vi "Configure DAQmx Task.vi"(8 "error in (no error)":errorcluster, 9 "DAQmx Timing Settings In":T2, 10 "Trigger Settings In":T1={"Trigger Type"=enum."No Trigger", "Digital Start"={"Source"="", "Digital Start Trigger Edge"=0}, "Digital Pause"={"Source"="", "Digital Pause Trigger Pause When"=0}, "Digital Reference"={"Source"="", "Digital Start Trigger Edge"=0, "Digital Reference Pretrigger Samples"=0}, "Analog Start"={"Source"="", "Analog Slope"=0, "Analog Start Trigger Hysteresis"=0.0, "Analog Start Trigger Level"=0.0}, "Analog Pause"={"Source"="", "Analog Start Trigger Level"=0.0, "Analog Pause Trigger Pause When"=10093}, "Analog Reference"={"Source"="", "Slope"=10280, "Pretrigger Samples"=0, "Level"=0.0}, "Time Start"={"Select Time\nManually"=FALSE, "When"=timestamp(0 s since 1904-01-01)}} caption="Some parts are hidden" {"Time Start"."When" format="%<%x %.3X>T"; "Analog Reference"."Level" format="%0.2f"; "Analog Reference"."Slope" items=["Rising"=10280, "Falling"=10171]; "Analog Pause"."Analog Pause Trigger Pause When" items=["Above Level"=10093, "Below Level"=10107]; "Analog Pause"."Analog Start Trigger Level" format="%0.2f"; "Analog Start"."Analog Start Trigger Level" format="%0.2f"; "Analog Start"."Analog Start Trigger Hysteresis" format="%.2f"; "Analog Start"."Analog Slope" items=["Rising"=10280, "Falling"=10171]; "Digital Reference"."Digital Start Trigger Edge" items=["Rising"=10280, "Falling"=10171]; "Digital Pause"."Digital Pause Trigger Pause When" items=["High"=10192, "Low"=10214]; "Digital Start"."Digital Start Trigger Edge" items=["Rising"=10280, "Falling"=10171]}, 11 "HW Refnum In":string) -> (0 "error out":errorcluster, 1 "Trigger Settings Out":T1={"Trigger Type"=enum."No Trigger", "Digital Start"={"Source"="", "Digital Start Trigger Edge"=0}, "Digital Pause"={"Source"="", "Digital Pause Trigger Pause When"=0}, "Digital Reference"={"Source"="", "Digital Start Trigger Edge"=0, "Digital Reference Pretrigger Samples"=0}, "Analog Start"={"Source"="", "Analog Slope"=0, "Analog Start Trigger Hysteresis"=0.0, "Analog Start Trigger Level"=0.0}, "Analog Pause"={"Source"="", "Analog Start Trigger Level"=0.0, "Analog Pause Trigger Pause When"=10093}, "Analog Reference"={"Source"="", "Slope"=10280, "Pretrigger Samples"=0, "Level"=0.0}, "Time Start"={"Select Time\nManually"=FALSE, "When"=timestamp(0 s since 1904-01-01)}} caption="Some parts are hidden" {"Time Start"."When" format="%<%x %.3X>T"; "Analog Reference"."Level" format="%0.2f"; "Analog Reference"."Slope" items=["Rising"=10280, "Falling"=10171]; "Analog Pause"."Analog Pause Trigger Pause When" items=["Above Level"=10093, "Below Level"=10107]; "Analog Pause"."Analog Start Trigger Level" format="%0.2f"; "Analog Start"."Analog Start Trigger Level" format="%0.2f"; "Analog Start"."Analog Start Trigger Hysteresis" format="%.2f"; "Analog Start"."Analog Slope" items=["Rising"=10280, "Falling"=10171]; "Digital Reference"."Digital Start Trigger Edge" items=["Rising"=10280, "Falling"=10171]; "Digital Pause"."Digital Pause Trigger Pause When" items=["High"=10192, "Low"=10214]; "Digital Start"."Digital Start Trigger Edge" items=["Rising"=10280, "Falling"=10171]}, 2 "DAQmx Timing Settings Out":T2, 3 "HW Refnum Out":string)   [LabVIEW 2020, in "Acquisition.lvlib"]
uses:
  Acquisition.lvlib
  Settings Editor/DAQmx Trigger Settings--cluster.ctl
  <vilib>/DAQmx/configure/timing.llb/DAQmx Timing (Sample Clock).vi
  <vilib>/DAQmx/configure/trigger.llb/DAQmx Start Trigger (Digital Edge).vi
  <vilib>/DAQmx/configure/trigger.llb/DAQmx Start Trigger (Time).vi
  <vilib>/DAQmx/configure/trigger.llb/DAQmx Start Trigger (Analog Edge).vi
  <vilib>/DAQmx/configure/trigger.llb/DAQmx Reference Trigger (Digital Edge).vi
  <vilib>/DAQmx/configure/trigger.llb/DAQmx Reference Trigger (Analog Edge).vi
  <resource>/objmgr/daqmx.rc
  Settings Editor/Settings Editor.lvlib
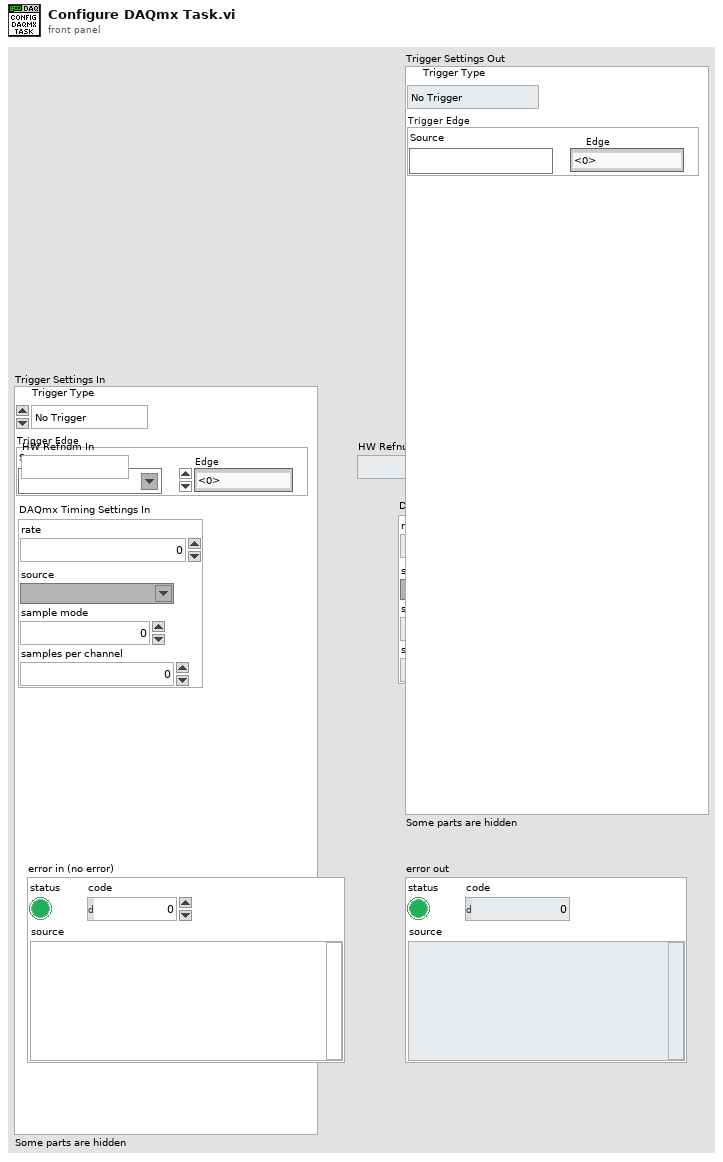
[diagram p1: front panel]
types:
  T1 = typedef "Settings Editor.lvlib/DAQmx Trigger Settings--cluster.ctl" = cluster{"Trigger Type":enum32{"No Trigger", "Digital Start", "Digital Pause", "Digital Reference", "Analog Start", "Analog Pause", "Analog Reference", "Time Start"}, "Digital Start":cluster{"Source":tag, "Digital Start Trigger Edge":i32}, "Digital Pause":cluster{"Source":tag, "Digital Pause Trigger Pause When":i32}, "Digital Reference":cluster{"Source":tag, "Digital Start Trigger Edge":i32, "Digital Reference Pretrigger Samples":u32}, "Analog Start":cluster{"Source":string, "Analog Slope":i32, "Analog Start Trigger Hysteresis":dbl, "Analog Start Trigger Level":dbl}, "Analog Pause":cluster{"Source":string, "Analog Start Trigger Level":dbl, "Analog Pause Trigger Pause When":i32}, "Analog Reference":cluster{"Source":string, "Slope":i32, "Pretrigger Samples":u32, "Level":dbl}, "Time Start":cluster{"Select Time\nManually":bool, "When":timestamp}}
  T2 = cluster{"rate":dbl, "source":tag, "sample mode":i32, "samples per channel":i32}
  T3 = enum32{"No Trigger", "Digital Start", "Digital Pause", "Digital Reference", "Analog Start", "Analog Pause", "Analog Reference", "Time Start"}
  T4 = cluster{"Source":tag, "Digital Start Trigger Edge":i32}
  T5 = cluster{"Select Time\nManually":bool, "When":timestamp}
  T6 = cluster{"Source":string, "Analog Slope":i32, "Analog Start Trigger Hysteresis":dbl, "Analog Start Trigger Level":dbl}
  T7 = cluster{"Source":tag, "Digital Start Trigger Edge":i32, "Digital Reference Pretrigger Samples":u32}
  T8 = cluster{"Source":string, "Slope":i32, "Pretrigger Samples":u32, "Level":dbl}
  T9 = cluster{"Source":tag, "Digital Pause Trigger Pause When":i32}
  T10 = cluster{"Source":string, "Analog Start Trigger Level":dbl, "Analog Pause Trigger Pause When":i32}
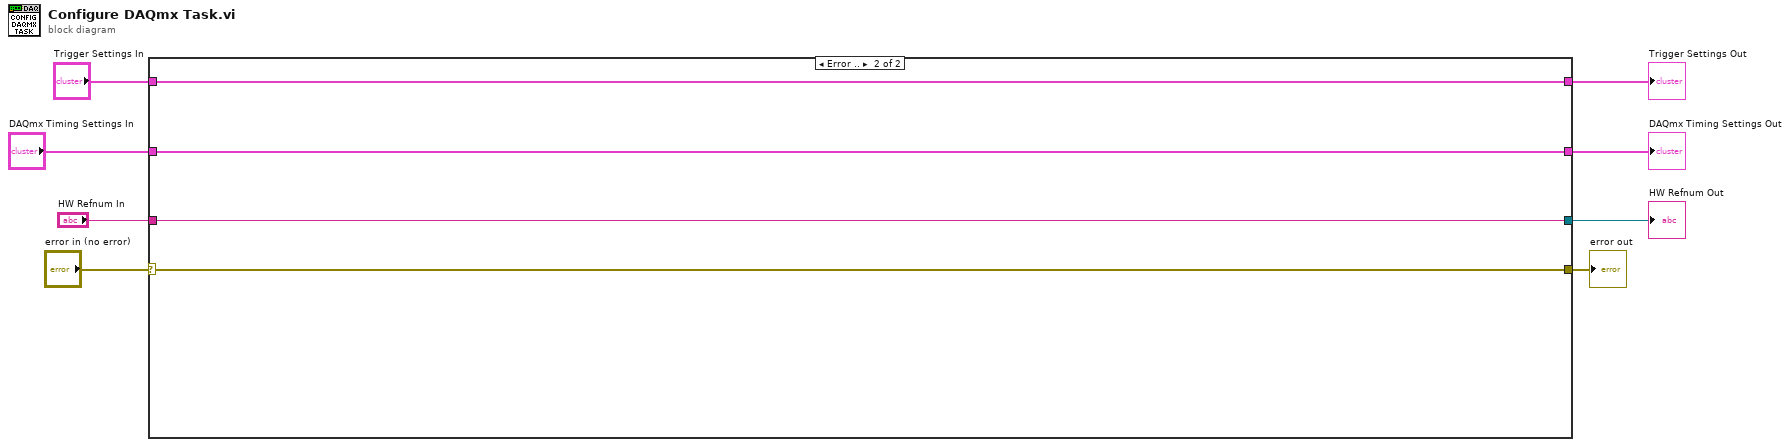
[diagram p0: block diagram]
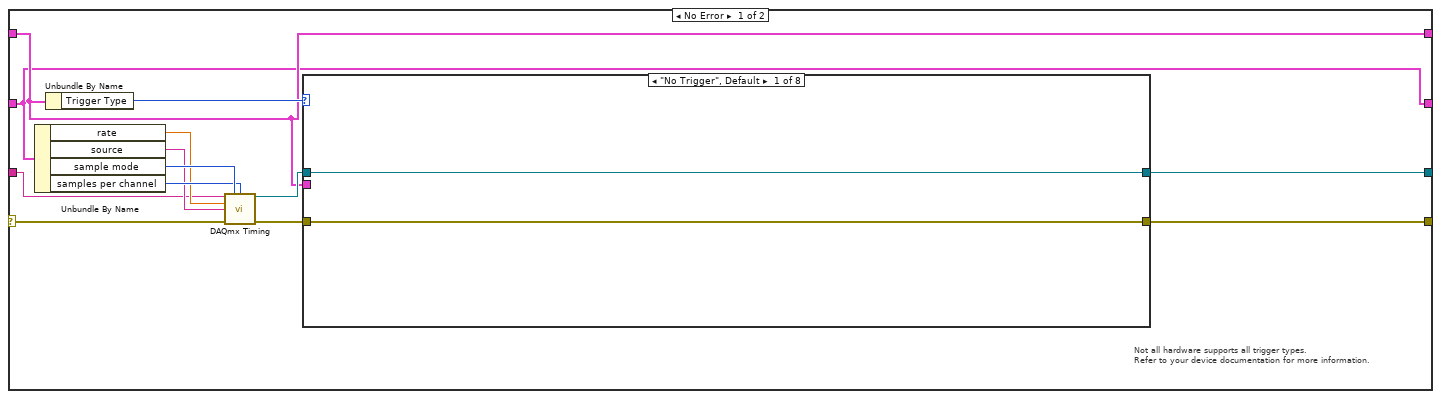
[diagram p2: hidden frame]
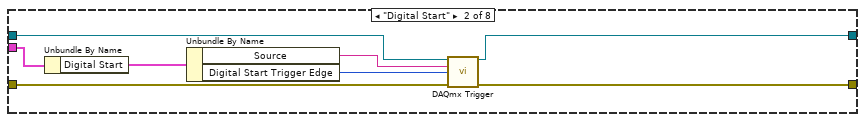
[diagram p3: hidden frame]
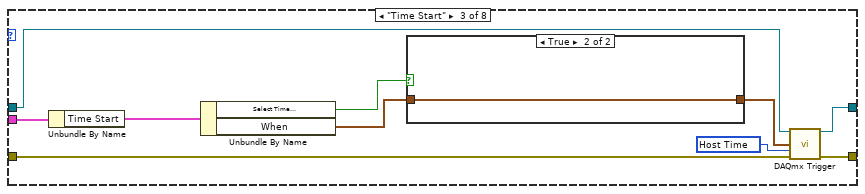
[diagram p4: hidden frame]
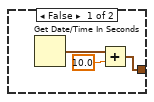
[diagram p5: hidden frame]
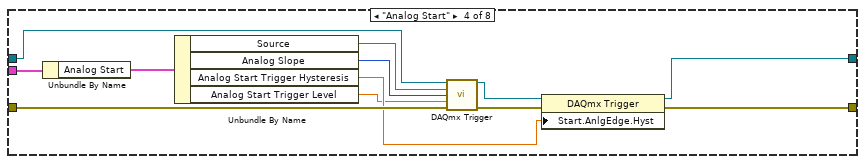
[diagram p6: hidden frame]
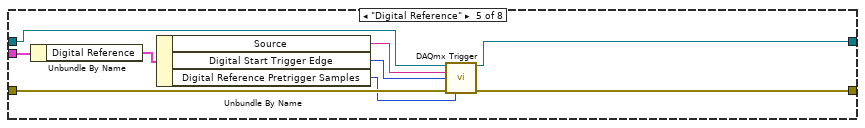
[diagram p7: hidden frame]
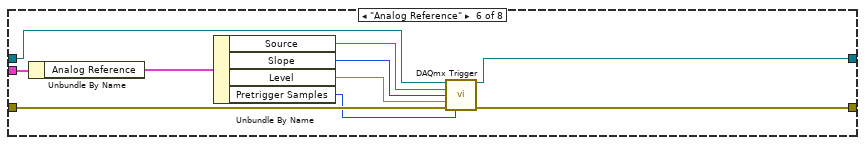
[diagram p8: hidden frame]
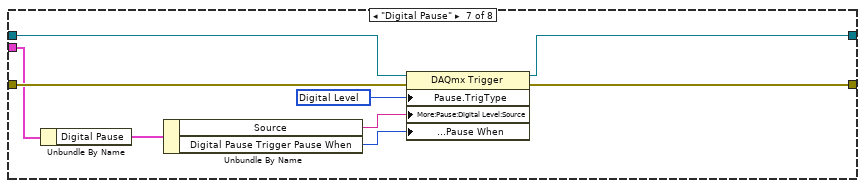
[diagram p9: hidden frame]
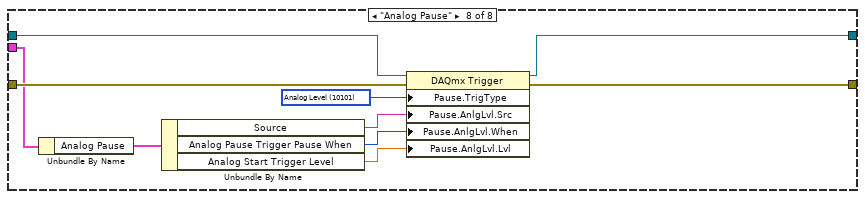
[diagram p10: hidden frame]
diagram:
  n1 = case shown="Error .." "error in (no error)" {
    selector: "error in (no error)" -> [w12 w98]
    tunnel: "DAQmx Timing Settings In" -> [w9 w96]
    tunnel: [w16 w99] -> w7
    tunnel: [w14 w98] -> w6
    tunnel: "Trigger Settings In" -> [w11 w97]
    tunnel: "HW Refnum In" -> [w10 w99]
    tunnel: [w11 w97] -> w2
    tunnel: [w9 w96] -> w1
    frame No Error {
      # "Not all hardware supports all trigger types.\nRefer to your device documentation for more information."
      n2 = Unbundle By Name(w9) -> ("rate"=w17:dbl, "source"=w18:tag, "sample mode"=w20:i32, "samples per channel"=w19:i32)
      n3 = Unbundle By Name(w11) -> ("Trigger Type"=w21:T3)
      n4 = call-poly <vilib>:"DAQmx Timing.vi"("task/channels in"=w10, "sample mode"=w20, "samples per channel"=w19, "rate"=w17, "source"=w18, "error in"=w12) -> ("task out"=w15:refnum<k21>, "error out"=w13:errorcluster)  [unwired: 8 in]
      n5 = case shown="\"No Trigger\", Default" w21 {
        tunnel: w15 -> [w23 w31 w36 w57 w66 w76 w85 w95]
        tunnel: [w23 w30 w41 w56 w65 w75 w84 w94] -> w16
        tunnel: [w22 w29 w40 w55 w64 w74 w83 w93] -> w14
        tunnel: w13 -> [w22 w28 w37 w52 w63 w73 w81 w92]
        tunnel: w11 -> [_ w25 w33 w47 w59 w68 w78 w87]
        frame "No Trigger", Default {
        }
        frame "Digital Start" {
          n6 = Unbundle By Name(w25) -> ("Digital Start"=w24:T4)
          n7 = Unbundle By Name(w24) -> ("Source"=w27:tag, "Digital Start Trigger Edge"=w26:i32)
          n8 = call-poly <vilib>:"DAQmx Trigger.vi"("task/channels in"=w31, "source"=w27, "edge"=w26, "error in"=w28) -> ("task out"=w30:refnum<k21>, "error out"=w29:errorcluster)  [unwired: 10 in]
        }
        frame "Time Start" {
          w39 = 16126 items=["Host Time"=16126, "I/O Device Time"=16127] ("timescale")
          n9 = Unbundle By Name(w33) -> ("Time Start"=w32:T5)
          n10 = Unbundle By Name(w32) -> ("Select Time\nManually"=w35:bool, "When"=w34:timestamp)
          n11 = case shown="True" w35 {
            tunnel: [w43 w45] -> w38
            tunnel: w34 -> [_ w45]
            frame False {
              n12 = Get Date/Time In Seconds() -> (seconds since 1Jan1904=w44:timestamp)
              n13 = Add(x=w44, y=10.0) -> (x+y=w43:timestamp)
            }
            frame True {
            }
          }
          n14 = call-poly <vilib>:"DAQmx Trigger.vi"("task/channels in"=w36, "when"=w38, "timescale"=w39, "error in"=w37) -> ("task out"=w41:refnum<k21>, "error out"=w40:errorcluster)  [unwired: 10 in]
        }
        frame "Analog Start" {
          n15 = Unbundle By Name(w47) -> ("Analog Start"=w46:T6)
          n16 = Unbundle By Name(w46) -> ("Source"=w51:string, "Analog Slope"=w50:i32, "Analog Start Trigger Hysteresis"=w49:dbl, "Analog Start Trigger Level"=w48:dbl)
          n17 = call-poly <vilib>:"DAQmx Trigger.vi"("task/channels in"=w57, "source"=w51, "slope"=w50, "level"=w48, "error in"=w52) -> ("task out"=w54:refnum<k21>, "error out"=w53:errorcluster)  [unwired: 9 in]
          n18 = property class="DAQmx Trigger"(reference=w54, error in=w53, "Start.AnlgEdge.Hyst"=w49) -> (reference out=w56:refnum<k21>, error out=w55:errorcluster)
        }
        frame "Digital Reference" {
          n19 = Unbundle By Name(w59) -> ("Digital Reference"=w58:T7)
          n20 = Unbundle By Name(w58) -> ("Source"=w62:tag, "Digital Start Trigger Edge"=w61:i32, "Digital Reference Pretrigger Samples"=w60:u32)
          n21 = call-poly <vilib>:"DAQmx Trigger.vi"("task/channels in"=w66, "source"=w62, "edge"=w61, "error in"=w63, "pretrigger samples per channel"=w60) -> ("task out"=w65:refnum<k21>, "error out"=w64:errorcluster)  [unwired: 9 in]
        }
        frame "Analog Reference" {
          n22 = Unbundle By Name(w68) -> ("Analog Reference"=w67:T8)
          n23 = Unbundle By Name(w67) -> ("Source"=w72:string, "Slope"=w71:i32, "Level"=w70:dbl, "Pretrigger Samples"=w69:u32)
          n24 = call-poly <vilib>:"DAQmx Trigger.vi"("task/channels in"=w76, "source"=w72, "slope"=w71, "level"=w70, "error in"=w73, "pretrigger samples per channel"=w69) -> ("task out"=w75:refnum<k21>, "error out"=w74:errorcluster)  [unwired: 8 in]
        }
        frame "Digital Pause" {
          w82 = 10152 items=["Analog Level"=10101, "Analog Window"=10103, "Digital Level"=10152, "Digital Pattern"=10398, "None"=10230] ("Pause.TrigType")
          n25 = Unbundle By Name(w78) -> ("Digital Pause"=w77:T9)
          n26 = Unbundle By Name(w77) -> ("Source"=w80:tag, "Digital Pause Trigger Pause When"=w79:i32)
          n27 = property class="DAQmx Trigger"(reference=w85, error in=w81, "Pause.TrigType"=w82, "More:Pause:Digital Level:Source"=w80, "More:Pause:Digital Level:Pause When"=w79) -> (reference out=w84:refnum<k21>, error out=w83:errorcluster)
        }
        frame "Analog Pause" {
          w91 = 10101 items=["Analog Level"=10101, "Analog Window"=10103, "Digital Level"=10152, "Digital Pattern"=10398, "None"=10230] ("Pause.TrigType")
          n28 = Unbundle By Name(w87) -> ("Analog Pause"=w86:T10)
          n29 = Unbundle By Name(w86) -> ("Source"=w90:string, "Analog Pause Trigger Pause When"=w89:i32, "Analog Start Trigger Level"=w88:dbl)
          n30 = property class="DAQmx Trigger"(reference=w95, error in=w92, "Pause.TrigType"=w91, "Pause.AnlgLvl.Src"=w90, "Pause.AnlgLvl.When"=w89, "Pause.AnlgLvl.Lvl"=w88) -> (reference out=w94:refnum<k21>, error out=w93:errorcluster)
        }
      }
    }
    frame Error {
    }
  }
  "HW Refnum Out" <- w7
  "error out" <- w6
  "Trigger Settings Out" <- w2
  "DAQmx Timing Settings Out" <- w1
